vi "MATLAB.vi"(11 "Graph":refnum<vi>) -> (0 "error out":errorcluster)   [LabVIEW 2022 SP3]
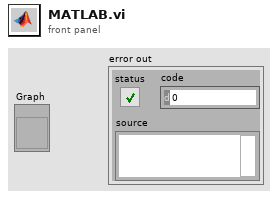
[diagram p1: front panel]
types:
  T1 = typedef "LVRangeTypeDef.ctl" = cluster{"Minimum":dbl, "Maximum":dbl, "Increment":dbl, "Minor Increment":dbl, "Start":dbl}
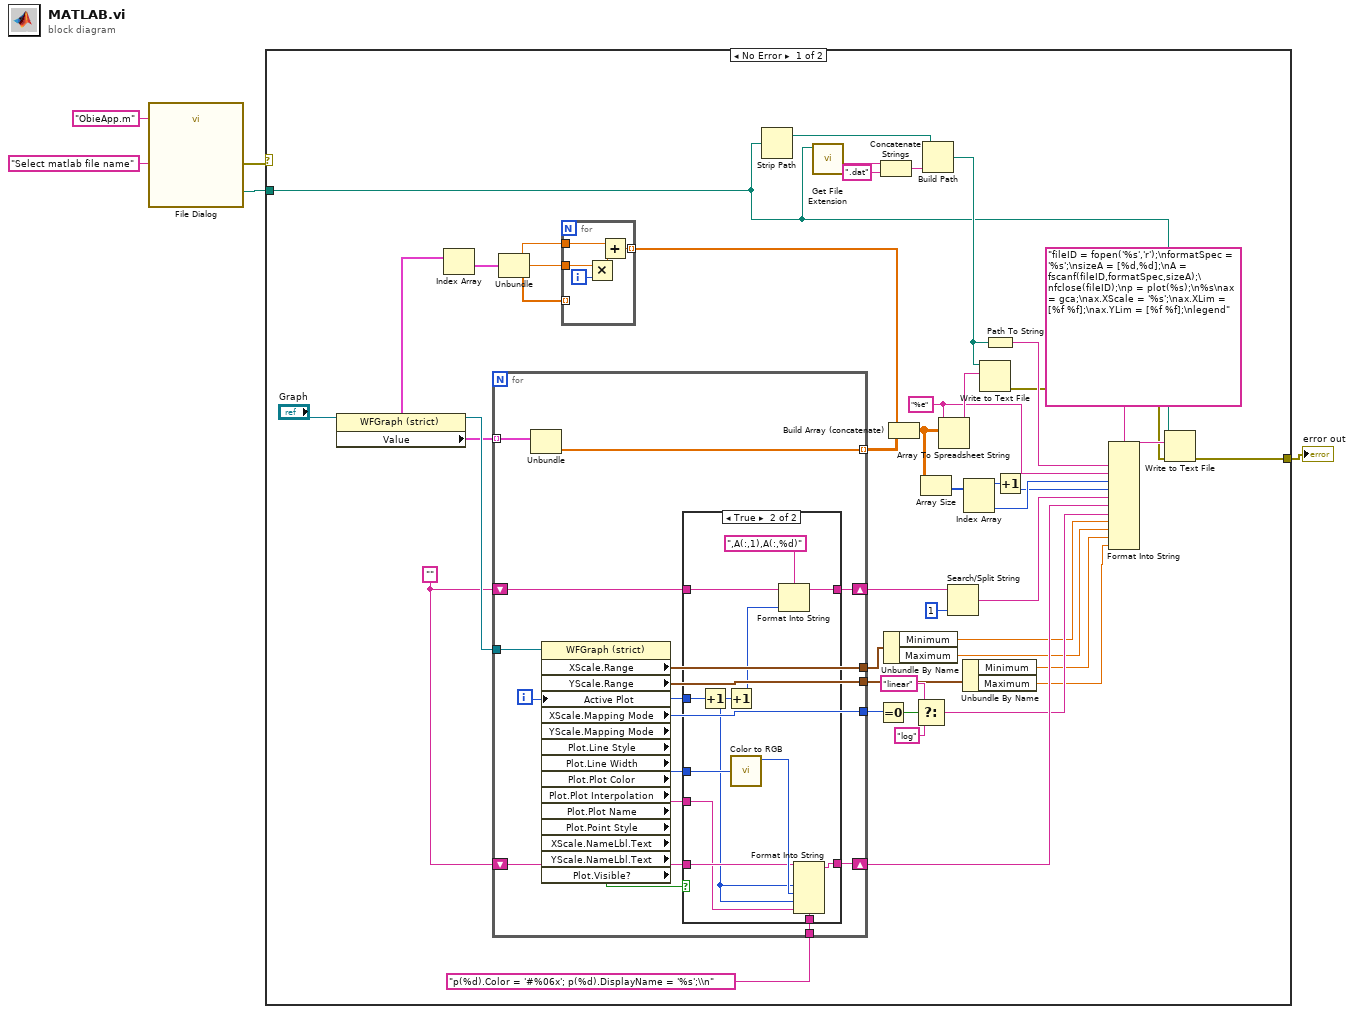
[diagram p0: block diagram]
diagram:
  n1 = call "File Dialog"("prompt"="Select matlab file name", "default name"="ObieApp.m") -> ("selected path"=w3:path, "error out"=w1:errorcluster)  [unwired: 10 in, 2 out]
  n2 = case shown="No Error" w1 {
    tunnel: w3 -> [w8 _]
    tunnel: [w6 _] -> w2
    frame No Error {
      w42 = "%e" ("format string")
      w33 = ""
      n3 = property class="WFGraph (strict)"(reference="Graph") -> (reference out=w48:refnum<vi>, "Value"=w19:cluster{dbl, "dt":dbl, "Y":dbl[]}[])  [unwired: 1 in, 1 out]
      n4 = Index Array(array=w19) -> (element=w18:cluster{dbl, "dt":dbl, "Y":dbl[]})  [unwired: 1 in]
      n5 = for {
        tunnel: w19 -> [w69] mode=indexing
        tunnel: w48 -> [w68]
        tunnel: [w56] -> w47 mode=indexing
        shift-right: [w64] -> w36
        shift-left: w33 -> [w65]
        shift-right: [w62] -> w32
        shift-left: w33 -> [w63]
        tunnel: "p(%d).Color = '#%06x'; p(%d).DisplayName = '%s';\\n" ("format string") -> [w61]
        tunnel: [w59] -> w30
        tunnel: [w58] -> w25
        tunnel: [w57] -> w23
        i -> [w66]
        n6 = Unbundle(w69) -> ("Y"=w56:dbl[])  [unwired: 2 out]
        n7 = property class="WFGraph (strict)" props=["XScale", "Range", "YScale", "Range", "Active Plot", "XScale", "Mapping Mode", "YScale", "Mapping Mode", "Plot", "Line Style", "Plot", "Line Width", "Plot", "Plot Color", "Plot", "Plot Interpolation", "Plot", "Plot Name", "Plot", "Point Style", "XScale", "NameLbl", "Text", "YScale", "NameLbl", "Text", "Plot", "Visible?"](reference=w68, "Active Plot"=w66) -> ("XScale.Range"=w58:T1, "YScale.Range"=w57:T1, "XScale.Mapping Mode"=w59:u8, "Plot.Plot Color"=w67:u32, "Plot.Plot Name"=w60:string, "Plot.Visible?"=w55:bool)  [unwired: 1 in, 9 out]
        n8 = case shown="True" w55 {
          tunnel: w67 -> [_ w83]
          tunnel: w66 -> [_ w81]
          tunnel: w65 -> [w71 w79]
          tunnel: [w71 w78] -> w64
          tunnel: w63 -> [w70 w76]
          tunnel: [w70 w75] -> w62
          tunnel: w61 -> [_ w74]
          tunnel: w60 -> [_ w72]
          frame False {
          }
          frame True {
            n9 = Increment(x=w81) -> (x+1=w73:i32)
            n10 = Increment(x=w73) -> (x+1=w80:i32)
            n11 = call <vilib>:"Color to RGB.vi"("Color"=w83) -> ("Resolved Color"=w77:u32)  [unwired: 3 out]
            n12 = Format Into String(format string=",A(:,1),A(:,%d)", initial string=w79, w80) -> (resulting string=w78:string)  [unwired: 1 in, 1 out]
            n13 = Format Into String(format string=w74, initial string=w76, w73, w77, w73, w72) -> (resulting string=w75:string)  [unwired: 1 in, 1 out]
          }
        }
      }
      n14 = Unbundle(w18) -> (w17:dbl, "dt"=w15:dbl, "Y"=w16:dbl[])
      n15 = for {
        tunnel: w16 -> [_] mode=indexing
        tunnel: w15 -> [w54]
        tunnel: w17 -> [w52]
        tunnel: [w51] -> w14 mode=indexing
        i -> [w50]
        n16 = Multiply(x=w54, y=w50) -> (x*y=w53:dbl)
        n17 = Add(x=w52, y=w53) -> (x+y=w51:dbl)
      }
      n18 = Strip Path(path=w8) -> (stripped path=w10:path)  [unwired: 1 out]
      n19 = call <vilib>:"Get File Extension.vi"("file"=w8) -> ("filename without extension"=w13:string)  [unwired: 6 in, 4 out]
      n20 = Equal To 0?(x=w30) -> (x = 0?=w29:bool)
      n21 = Concatenate Strings(w13, ".dat" ("string")) -> (w11:string)
      n22 = Unbundle By Name(w25) -> ("Minimum"=w24:dbl, "Maximum"=w22:dbl)
      n23 = Build Array (concatenate)(w14, w47) -> (w45:dbl[][])
      n24 = Select(t="linear", s=w29, f="log") -> (s? t:f=w26:string)
      n25 = Array Size(array=w45) -> (size(s)=w44:i32[])
      n26 = Build Path(base path=w10, name or relative path=w11) -> (appended path=w9:path)
      n27 = Array To Spreadsheet String(array=w45, 3:w42) -> (spreadsheet string=w46:string)  [unwired: 1 in]
      n28 = Search/Split String(string=w36, offset (0)=1) -> (match + rest of string=w35:string)  [unwired: 1 in, 2 out]
      n29 = Unbundle By Name(w23) -> ("Minimum"=w21:dbl, "Maximum"=w20:dbl)
      n30 = Index Array(array=w44) -> (element #1=w41:i32, element #2=w38:i32)  [unwired: 2 in]
      n31 = Write to Text File(file (use dialog)=w9, text=w46) -> (error out=w7:errorcluster)  [unwired: 2 in, 2 out]
      n32 = Path To String(path=w9) -> (string=w40:string)
      n33 = Increment(x=w41) -> (x+1=w37:i32)
      n34 = Format Into String(format string="fileID = fopen('%s','r');\nformatSpec = '%s';\nsizeA = [%d,%d];\nA = fscanf(fileID,formatSpec,sizeA);\nfclose(fileID);\np = plot(%s);\n%s\nax = gca;\nax.XScale = '%s';\nax.XLim = [%f %f];\nax.YLim = [%f %f];\nlegend", w40, w42, w38, w37, w35, w32, w26, w24, w22, w21, w20) -> (resulting string=w39:string)  [unwired: 2 in, 1 out]
      n35 = Write to Text File(file (use dialog)=w8, text=w39, error in=w7) -> (error out=w6:errorcluster)  [unwired: 1 in, 2 out]
    }
    frame Error {
    }
  }
  "error out" <- w2
